vi "Launcher.vi"() -> ()   [LabVIEW 2024]
uses:
  Implementations/Logger/Logger.lvclass
  C:/Users/burakkorkmaz/Desktop/Leveling/labview-desing-patterns/Bridge Pattern/IDataMethod_interface/IDataMethod.lvclass
  Implementations/Viewer/Viewer.lvclass
  Abstractions/TDMS/TDMS.lvclass
  Support/Type Def/Requirements.ctl
  <vilib>/numeric/Random Number (Range) DBL.vi
  Support/Type Def/Data.ctl
  <vilib>/Utility/file.llb/Write Delimited Spreadsheet (string).vi
  C:/Users/burakkorkmaz/Desktop/Leveling/labview-desing-patterns/Bridge Pattern/Implementations/Logger/Logger.lvclass
  C:/Users/burakkorkmaz/Desktop/Leveling/labview-desing-patterns/Bridge Pattern/Implementations/Viewer/Viewer.lvclass
panel:
  in  "File Method":enum32{"Item 0", "Item 1"}(radio)
  in  "File Type":enum32{"Item 0", "Item 1"}(radio)
  in  "Tab Control":enum32{"LOG", "VIEW"}(tab)
  in  "LogData":cluster{"Speed":dbl, "Torque":dbl}
  in  "Log Button":bool
  in  "Log History":string[][](table)
  in  "File View":string[][](table)
  in  "Reflesh Rate":dbl
  # "Made by Ramazan Burak Korkmaz"
  # "DATA"
  # "LOG HISTORY"
  # "Speed"
  # "Torque"
  # "DATA"
  # "Speed"
  # "Torque"
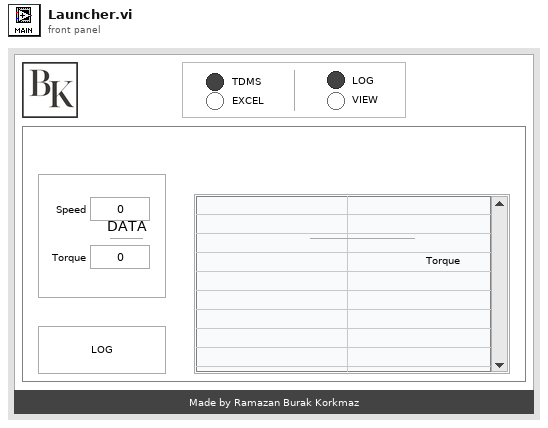
[diagram p1: front panel]
types:
  T1 = typedef "Data.ctl" = map{string, dbl[]}
  T2 = enum16{"open", "open or create", "create or replace", "create", "open (read-only)"}
  T3 = typedef "Requirements.ctl" = cluster{"From":enum16{"TDMS", "EXCEL"}, "File Handler":variant, "Input":variant}
  T4 = typedef "Message.ctl" = cluster{"Message":string, "From":enum16{"LOGGER", "VIEWER"}, "Return":variant}
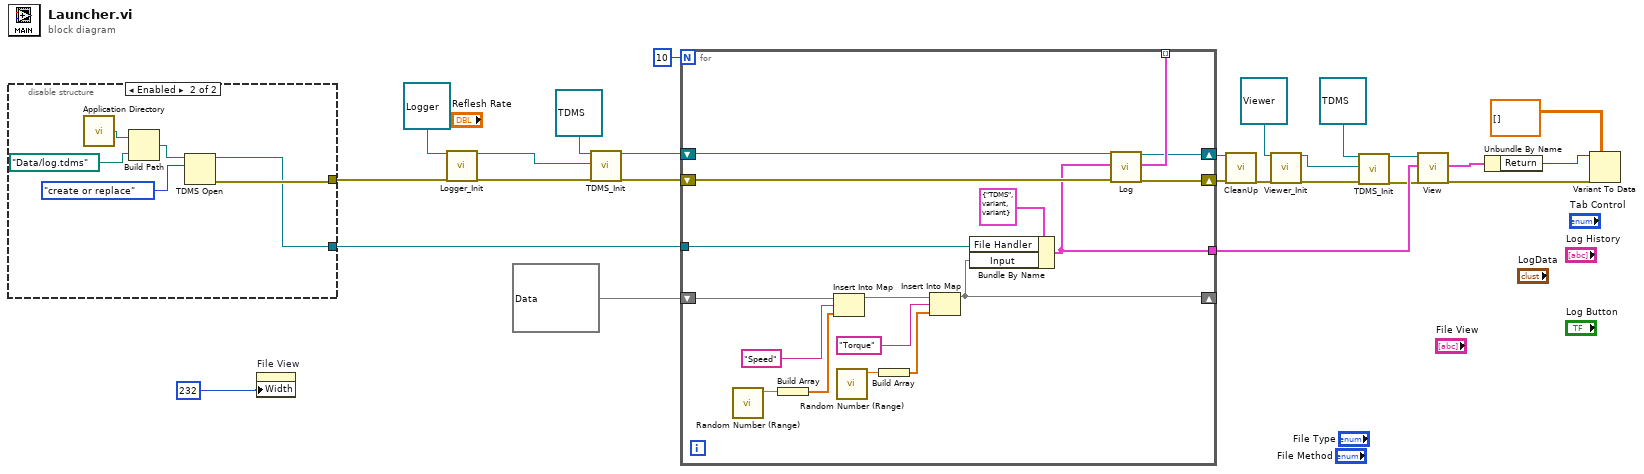
[diagram p0: block diagram]
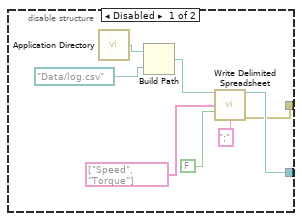
[diagram p2: hidden frame]
diagram:
  n1 = disable-structure shown="Enabled" {
    disable-tunnel: [w31 w41] -> w28
    disable-tunnel: [w29 w42] -> w25
    frame Disabled {
      n2 = call <vilib>:"Application Directory.vi"() -> ("Application Directory"=w36:path)
      n3 = Build Path(base path=w36, name or relative path=path "Data/log.csv") -> (appended path=w34:path)
      n4 = call-poly <vilib>:"Write Delimited Spreadsheet.vi"("file path (dialog if empty)"=w34, "1D data"=string[] ["Speed", "Torque"], "append to file? (new file:F)"=FALSE, "delimiter (\\t)"=";" ("delimiter (\\t)")) -> ("new file path (Not A Path if cancelled)"=w31:path, "error out"=w29:errorcluster)  [unwired: 10 in]
    }
    frame Enabled {
      n5 = call <vilib>:"Application Directory.vi"() -> ("Application Directory"=w39:path)
      n6 = Build Path(base path=w39, name or relative path=path "Data/log.tdms") -> (appended path=w38:path)
      n7 = TDMS Open(10:T2."create or replace" ("operation (0:open)"), 11:w38) -> (0:w42:errorcluster, 3:w41:refnum<k34>)  [unwired: 5 in]
    }
  }
  n8 = property on="File View" class="Tbl (strict)"("Width"=u32 232 ("Active Cell:Cell Size:Width")) -> ()  [unwired: 2 in, 2 out]
  n9 = call "Logger_Init.vi"("object in"=refnum<class "Logger.lvclass"> refnum ("Logger"), "error in (no error)"=w25) -> ("object out"=w20:refnum<class "Logger.lvclass">, "error out"=w19:errorcluster)  [unwired: 16 in]
  n10 = call "TDMS_Init.vi"("object in"=refnum<class "TDMS.lvclass"> refnum ("TDMS"), "Data Method"=w20, "error in (no error)"=w19) -> ("object out"=w23:refnum<class "TDMS.lvclass">, "error out"=w22:errorcluster)  [unwired: 15 in]
  n11 = for {
    N: 10 -> [_]
    tunnel: w28 -> [w56]
    shift-right: [w47] -> w11
    shift-left: w22 -> [w58]
    shift-right: [w46] -> w10
    shift-left: w23 -> [w59]
    tunnel: [w48] -> w26 mode=indexing
    tunnel: [w45] -> w18
    shift-right: [w43] -> w2
    shift-left: T1 {} ("Data") -> [w44]
    n12 = call-poly <vilib>:"Random Number (Range).vi"() -> ("number"=w55:dbl)  [unwired: 11 in]
    n13 = Build Array(w55) -> (w54:dbl[])
    n14 = Insert Into Map(map in=w44, key="Speed", value=w54) -> (map out=w52:T1)  [unwired: 2 out]
    n15 = call-poly <vilib>:"Random Number (Range).vi"() -> ("number"=w50:dbl)  [unwired: 11 in]
    n16 = Build Array(w50) -> (w49:dbl[])
    n17 = Insert Into Map(map in=w52, key="Torque", value=w49) -> (map out=w43:T1)  [unwired: 2 out]
    n18 = Bundle By Name(cluster=T3 {"From"=enum."TDMS", "File Handler"=variant, "Input"=variant} ("Requirements"), "File Handler"=w56, "Input"=w43) -> (w45:T3)
    n19 = call-dynamic "Log.vi"("object in"=w59, "Requirements"=w45, "Error In"=w58) -> ("object out"=w46:refnum<class "TDMS.lvclass">, "Message"=w48:T4, "Error Out"=w47:errorcluster)  [unwired: 14 in]
  }
  n20 = call-dynamic "CleanUp.vi"("object in"=w10, "error in (no error)"=w11) -> ("error out"=w4:errorcluster)  [unwired: 16 in, 1 out]
  n21 = call "Viewer_Init.vi"("object in"=refnum<class "Viewer.lvclass"> refnum ("Viewer"), "error in (no error)"=w4) -> ("object out"=w6:refnum<class "Viewer.lvclass">, "error out"=w9:errorcluster)  [unwired: 16 in]
  n22 = call "TDMS_Init.vi"("object in"=refnum<class "TDMS.lvclass"> refnum ("TDMS"), "Data Method"=w6, "error in (no error)"=w9) -> ("object out"=w7:refnum<class "TDMS.lvclass">, "error out"=w8:errorcluster)  [unwired: 15 in]
  n23 = call-dynamic "View.vi"("object in"=w7, "Requirements"=w18, "Error In"=w8) -> ("Message"=w13:T4, "Error Out"=w16:errorcluster)  [unwired: 14 in, 1 out]
  n24 = Unbundle By Name(w13) -> ("Return"=w17:variant)
  n25 = Variant To Data(error in=w16, type=dbl[][] [], Variant=w17) -> (data=w14:dbl[][])  [unwired: 1 out]
